vi "monitor.vi"() -> ()   [LabVIEW 2012]
uses:
  <vilib>/addons/database/Auxilliary.llb/DB Tools Cursor Type.ctl
  <vilib>/addons/database/Connection.llb/DB Tools Open Connec (Path).vi
  <vilib>/addons/database/Connection.llb/Conn Execute.vi
  <vilib>/addons/database/Recordset.llb/Rec Fetch Recordset Data (R).vi
  <vilib>/addons/database/Recordset.llb/Rec Destroy - Connection.vi
  <vilib>/addons/database/_DB Variant To Data/Database Variant To Data.xnode
  <vilib>/addons/database/NI_Database_API.lvlib
panel:
  in  "Table Control":string[][](table)
  out "error out 2":errorcluster
  in  "input cluster 2":T1
  in  "stop":bool
  in  "OK Button":bool
  in  "M100 Monitor Board":string[][](table)
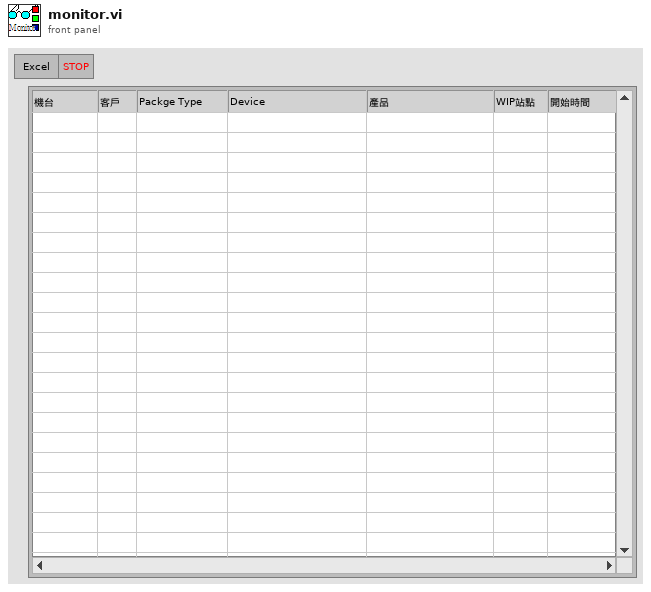
[diagram p1: front panel]
types:
  T1 = cluster{"Customer":string, "Package":string, "machine":string}
  T2 = typedef "NI_Database_API.lvlib/DB Tools Cursor Type.ctl" = enum16{"forward-only", "keyset", "dynamic", "static"}
  T3 = typedef "NI_Database_API.lvlib/Conn ObjectReference.ctl" = refnum<k1>
  T4 = typedef "LVDateTimeRec.ctl" = cluster{"fractional second":dbl, "second":i32, "minute":i32, "hour":i32, "day of month":i32, "month":i32, "year":i32, "day of week":i32, "day of year":i32, "DST":i32}
  T5 = typedef "LVRowAndColumnTypeDef.ctl" = cluster{"Row":i32, "Column":i32}
  T6 = typedef "NI_Database_API.lvlib/Rec ObjectReference.ctl" = refnum<k1>
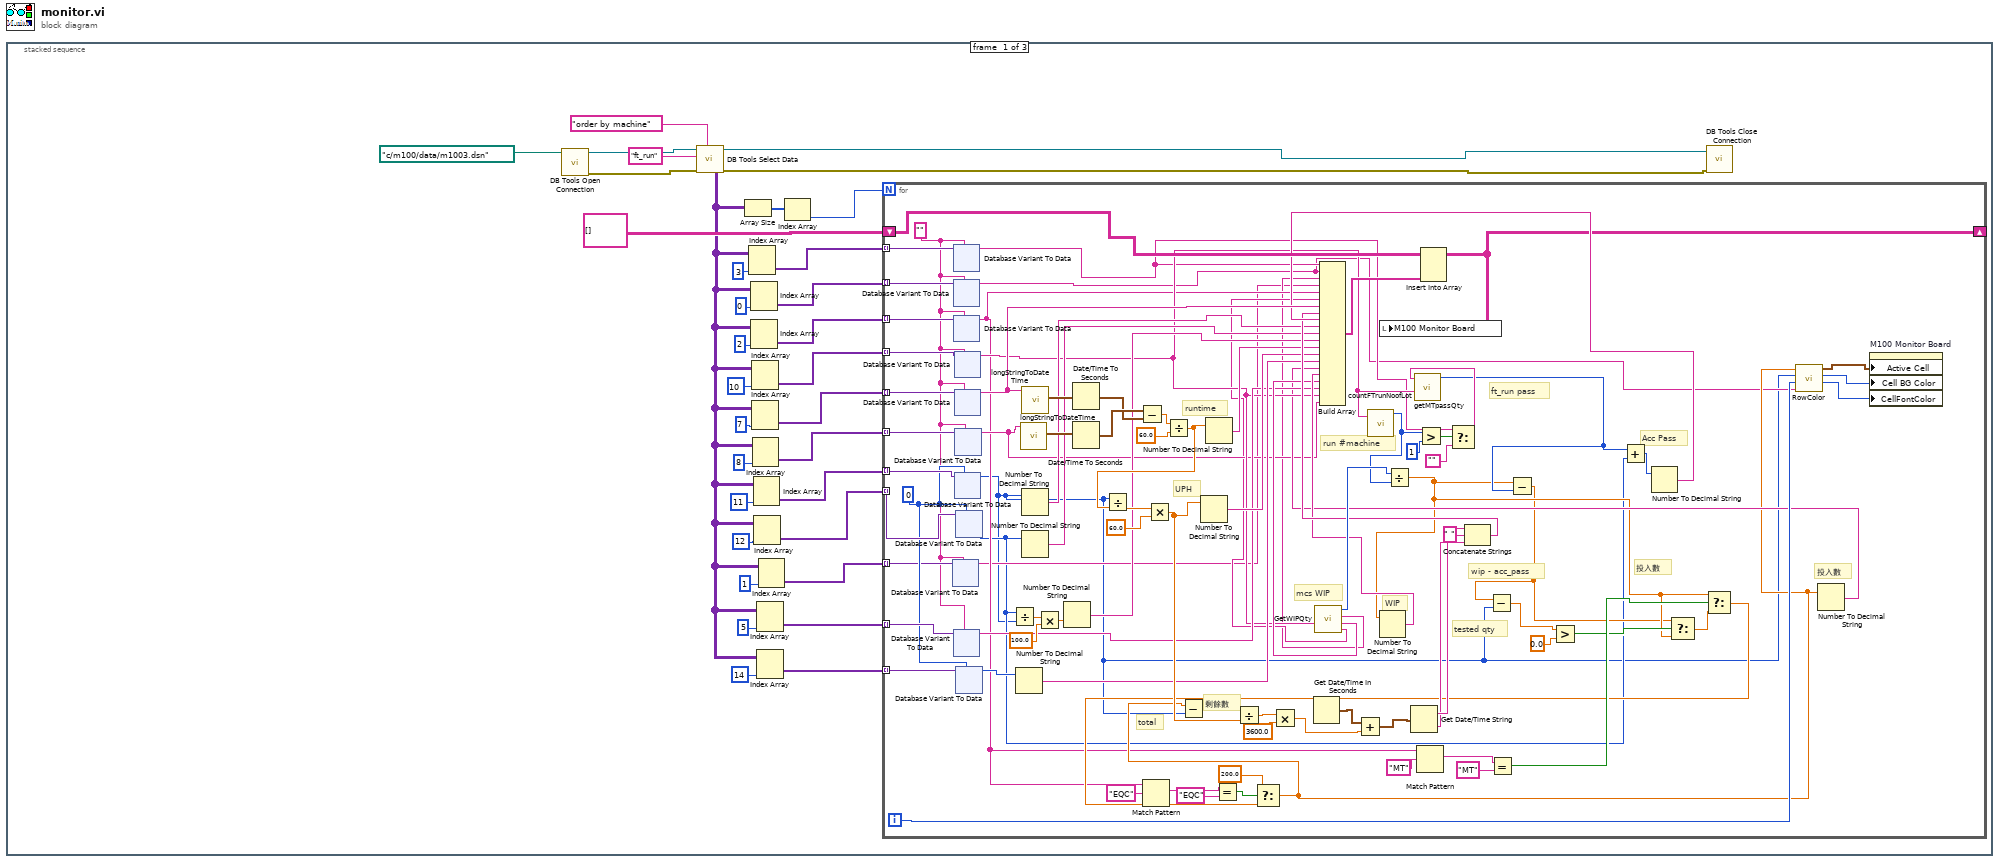
[diagram p0: block diagram]
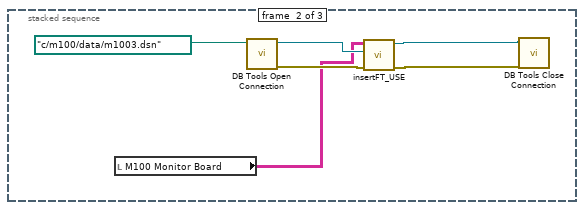
[diagram p2: hidden frame]
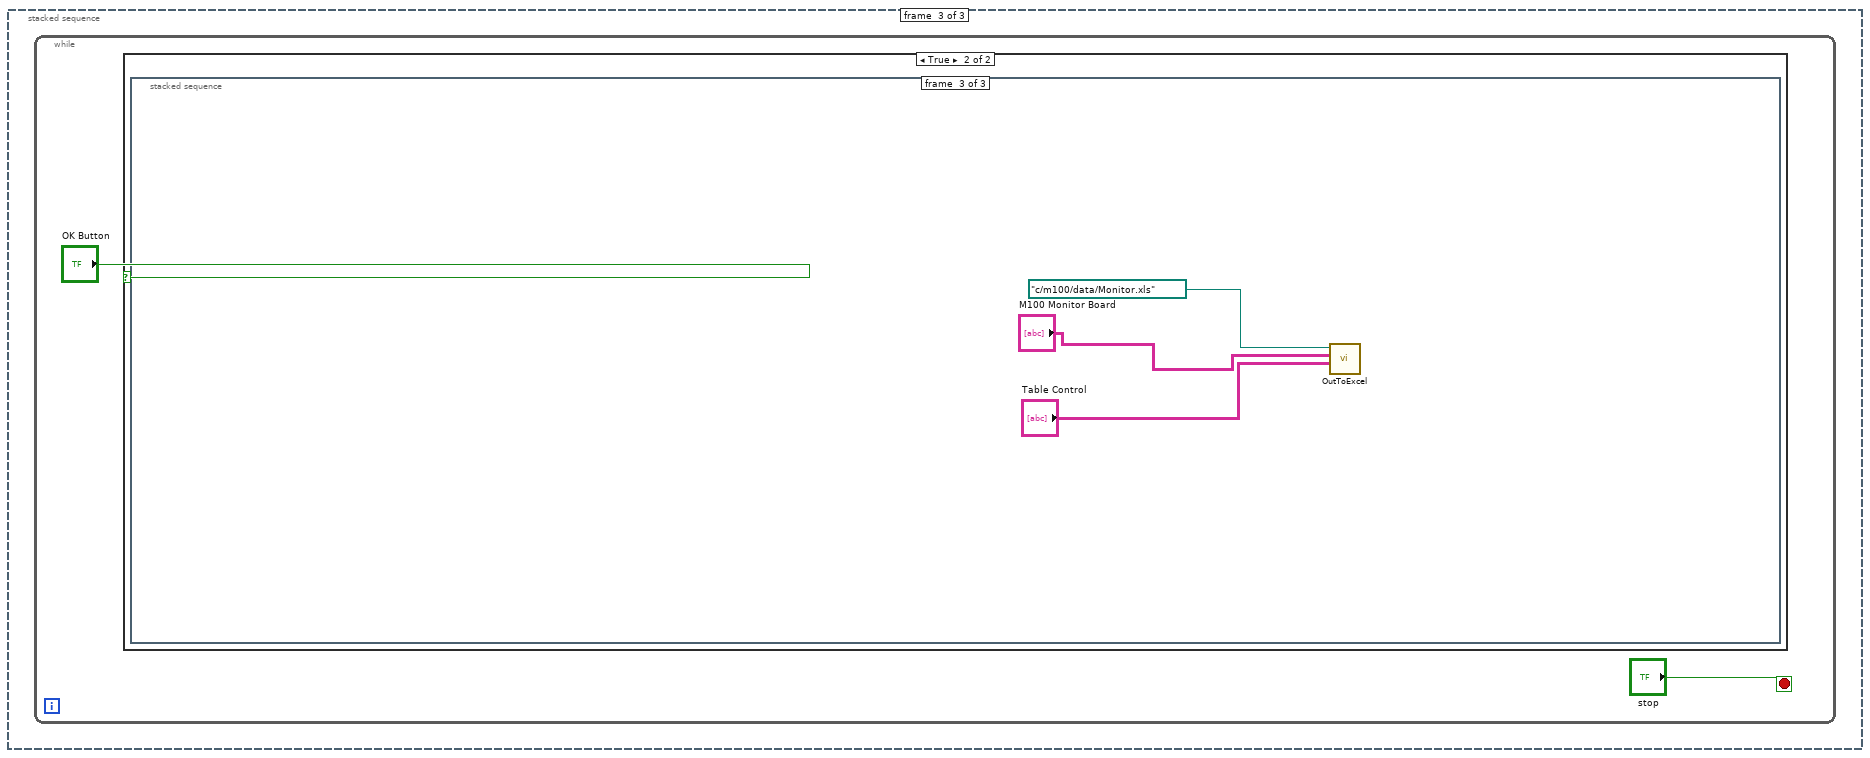
[diagram p3: hidden frame]
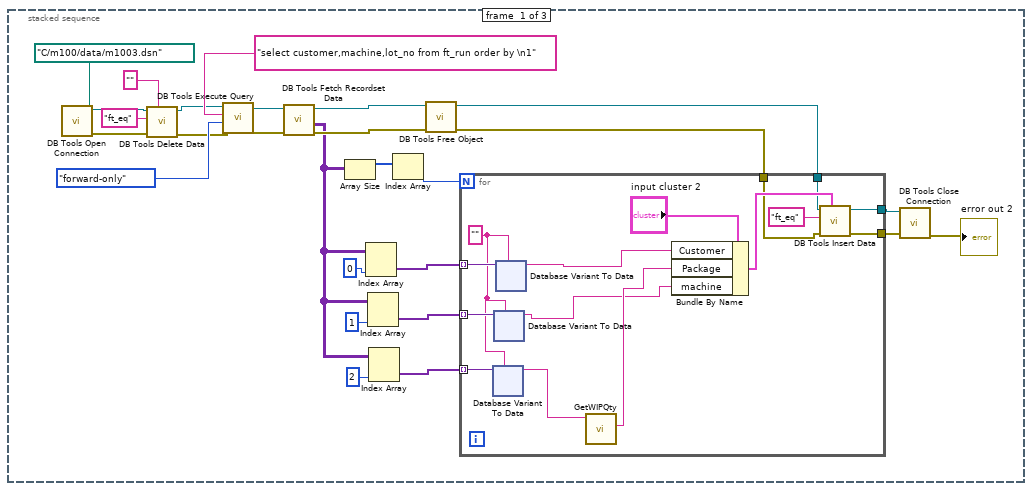
[diagram p5: hidden frame]
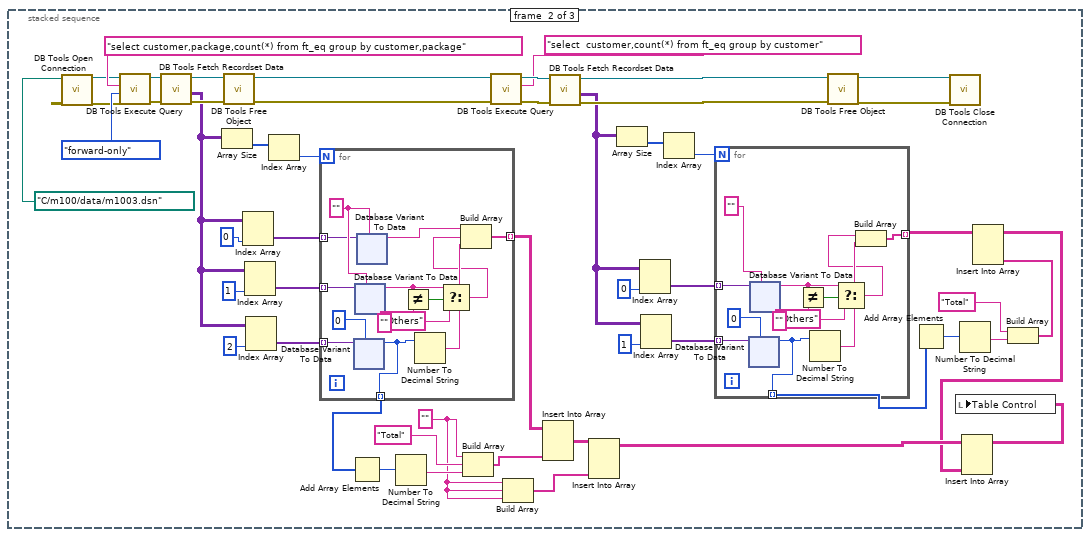
[diagram p6: hidden frame]
diagram:
  n1 = stacked-sequence {
    frame #0 {
      n2 = call-poly <vilib>:"DB Tools Open Connection.vi"("connection information"=path "c:/m100/data/m1003.dsn") -> ("error out"=w32:errorcluster, "connection reference"=w33:T3)  [unwired: 7 in]
      n3 = call <vilib>:"DB Tools Select Data.vi"("condition"="order by machine", "error in (no error)"=w32, "table"="ft_run", "connection reference"=w33) -> ("error out"=w1:errorcluster, "data"=w5:variant[][], "connection reference out"=w2:T3)  [unwired: 2 in]
      n4 = Array Size(array=w5) -> (size(s)=w29:i32[])
      n5 = Index Array(array=w5, index (col)=3) -> (element=w18:variant[])  [unwired: 1 in]
      n6 = Index Array(array=w5, index (col)=0) -> (element=w25:variant[])  [unwired: 1 in]
      n7 = Index Array(array=w5, index (col)=2) -> (element=w17:variant[])  [unwired: 1 in]
      n8 = Index Array(array=w5, index (col)=10) -> (element=w16:variant[])  [unwired: 1 in]
      n9 = Index Array(array=w5, index (col)=7) -> (element=w15:variant[])  [unwired: 1 in]
      n10 = Index Array(array=w5, index (col)=8) -> (element=w11:variant[])  [unwired: 1 in]
      n11 = Index Array(array=w5, index (col)=11) -> (element=w14:variant[])  [unwired: 1 in]
      n12 = Index Array(array=w5, index (col)=12) -> (element=w13:variant[])  [unwired: 1 in]
      n13 = Index Array(array=w5, index (col)=5) -> (element=w9:variant[])  [unwired: 1 in]
      n14 = Index Array(array=w5, index (col)=14 ("disabled index (col)")) -> (element=w7:variant[])  [unwired: 1 in]
      n15 = Index Array(array=w5, index (col)=1 ("disabled index (col)")) -> (element=w3:variant[])  [unwired: 1 in]
      n16 = Index Array(array=w29) -> (element=w28:i32)  [unwired: 1 in]
      n17 = for {
        N: w28 -> [_]
        tunnel: w25 -> [w120] mode=indexing
        tunnel: w13 -> [w124] mode=indexing
        shift-right: [w42] -> _
        shift-left: string[][] [] -> [w123]
        tunnel: w18 -> [w121] mode=indexing
        tunnel: w17 -> [w119] mode=indexing
        tunnel: w16 -> [w118] mode=indexing
        tunnel: w15 -> [w117] mode=indexing
        tunnel: w14 -> [w116] mode=indexing
        tunnel: w11 -> [w112] mode=indexing
        tunnel: w9 -> [w102] mode=indexing
        tunnel: w7 -> [w101] mode=indexing
        tunnel: w3 -> [w50] mode=indexing
        i -> [w86]
        w100 = 0
        w49 = ""
        # "tested qty"
        # "wip - acc_pass"
        # "投入數"
        # "剩餘數"
        # "ft_run pass"
        # "WIP"
        # "mcs WIP"
        # "run #machine"
        # "Acc Pass"
        # "total"
        # "UPH"
        # "runtime"
        # "投入數"
        n18 = xnode "Database Variant To Data"("database variant"=w50, "type"=w49) -> ("data"=w43:string)  [unwired: 1 in, 1 out]
        n19 = xnode "Database Variant To Data"("database variant"=w121, "type"=w49) -> ("data"=w46:string)  [unwired: 1 in, 1 out]
        n20 = xnode "Database Variant To Data"("database variant"=w120, "type"=w49) -> ("data"=w45:string)  [unwired: 1 in, 1 out]
        n21 = xnode "Database Variant To Data"("database variant"=w119, "type"=w49) -> ("data"=w48:string)  [unwired: 1 in, 1 out]
        n22 = xnode "Database Variant To Data"("database variant"=w102, "type"=w49) -> ("data"=w67:string)  [unwired: 1 in, 1 out]
        n23 = xnode "Database Variant To Data"("database variant"=w118, "type"=w49) -> ("data"=w66:string)  [unwired: 1 in, 1 out]
        n24 = xnode "Database Variant To Data"("database variant"=w117, "type"=w49) -> ("data"=w78:string)  [unwired: 1 in, 1 out]
        n25 = xnode "Database Variant To Data"("database variant"=w116, "type"=w100) -> ("data"=w34:i32)  [unwired: 1 in, 1 out]
        n26 = xnode "Database Variant To Data"("database variant"=w112, "type"=w49) -> ("data"=w63:string)  [unwired: 1 in, 1 out]
        n27 = xnode "Database Variant To Data"("database variant"=w124, "type"=w100) -> ("data"=w36:i32)  [unwired: 1 in, 1 out]
        n28 = xnode "Database Variant To Data"("database variant"=w101, "type"=w100) -> ("data"=w99:i32)  [unwired: 1 in, 1 out]
        n29 = Divide(x=w36, y=w34) -> (x/y=w113:dbl)
        n30 = Number To Decimal String(number=w99) -> (decimal integer string=w70:string)  [unwired: 1 in]
        n31 = call "longStringToDateTime.vi"("input string"=w63) -> ("output cluster"=w111:T4)  [unwired: 10 in]
        n32 = call "longStringToDateTime.vi"("input string"=w78) -> ("output cluster"=w110:T4)  [unwired: 10 in]
        n33 = Number To Decimal String(number=w34) -> (decimal integer string=w75:string)  [unwired: 1 in]
        n34 = Number To Decimal String(number=w36) -> (decimal integer string=w74:string)  [unwired: 1 in]
        n35 = Multiply(x=w113, y=100.0) -> (x*y=w114:dbl)
        n36 = Number To Decimal String(number=w114) -> (decimal integer string=w73:string)  [unwired: 1 in]
        n37 = Date/Time To Seconds(2:w110) -> (0:w108:timestamp)  [unwired: 1 in]
        n38 = Date/Time To Seconds(2:w111) -> (0:w109:timestamp)  [unwired: 1 in]
        n39 = Subtract(x=w109, y=w108) -> (x-y=w107:dbl)
        n40 = Match Pattern(string=w48, regular expression="EQC") -> (match substring=w61:string)  [unwired: 1 in, 3 out]
        n41 = Divide(x=w107, y=60.0) -> (x/y=w105:dbl)
        n42 = Divide(x=w34, y=w105) -> (x/y=w104:dbl)
        n43 = Multiply(x=w104, y=60.0) -> (x*y=w98:dbl)
        n44 = Number To Decimal String(number=w98) -> (decimal integer string=w71:string)  [unwired: 1 in]
        n45 = Number To Decimal String(number=w105) -> (decimal integer string=w72:string)  [unwired: 1 in]
        n46 = Equal?(x=w61, y="EQC") -> (x = y?=w59:bool)
        n47 = Get Date/Time In Seconds() -> (seconds since 1Jan1904=w95:timestamp)
        n48 = call "GetWIPQty.vi"("Lotno"=w66) -> ("step"=w47:string, "lotno"=w68:string, "Package"=w44:string, "data"=w85:i32)  [unwired: 7 in]
        n49 = call "countFTrunNoofLot.vi"("Lotno"=w66) -> ("data"=w83:i32)  [unwired: 10 in]
        n50 = Divide(x=w85, y=w83) -> (x/y=w39:dbl)
        n51 = Number To Decimal String(number=w39) -> (decimal integer string=w69:string)  [unwired: 1 in]
        n52 = Match Pattern(string=w48, regular expression="MT") -> (match substring=w56:string)  [unwired: 1 in, 3 out]
        n53 = Greater?(x=w83, y=1) -> (0:w81:bool)
        n54 = Select(t=w46, s=w81, f="") -> (s? t:f=w79:string)
        n55 = call "getMTpassQty.vi"("Lot"=w66, "machine"=w79) -> ("data"=w64:i32)  [unwired: 9 in]
        n56 = Equal?(x=w56, y="MT") -> (x = y?=w54:bool)
        n57 = Subtract(x=w39, y=w64) -> (x-y=w37:dbl)
        n58 = Subtract(x=w37, y=w34) -> (x-y=w35:dbl)
        n59 = Greater?(x=w35, y=0.0) -> (0:w40:bool)
        n60 = Add(x=w64, y=w36) -> (x+y=w84:i32)
        n61 = Number To Decimal String(number=w84) -> (decimal integer string=w77:string)  [unwired: 1 in]
        n62 = Select(t=w37, s=w40, f=w39) -> (s? t:f=w38:dbl)
        n63 = Select(t=w39, s=w54, f=w38) -> (s? t:f=w53:dbl)
        n64 = Select(t=200.0, s=w59, f=w53) -> (s? t:f=w51:dbl)
        n65 = Subtract(x=w51, y=w34) -> (x-y=w52:dbl)
        n66 = Divide(x=w52, y=w98) -> (x/y=w97:dbl)
        n67 = Multiply(x=w97, y=3600.0) -> (x*y=w94:dbl)
        n68 = Add(x=w95, y=w94) -> (x+y=w93:timestamp)
        n69 = Get Date/Time String(seconds (now)=w93) -> (date string=w92:string, time string=w91:string)  [unwired: 2 in]
        n70 = Concatenate Strings(w92, " " ("string"), w91) -> (w76:string)
        n71 = call "RowColor.vi"("Customer"=w45, "Row"=w86, "tested"=w34, "Input"=w51) -> ("FontColor"=w87:u32, "bgcolor"=w88:u32, "ActiveCell"=w89:T5)  [unwired: 5 in]
        n72 = Number To Decimal String(number=w51) -> (decimal integer string=w65:string)  [unwired: 1 in]
        n73 = Build Array(w46, w45, w44, w43, w48, w47, w78, w76, w77, w75, w74, w73, w72, w71, w70, w65, w69, w68, w67, w66, w63) -> (w122:string[])
        n74 = Insert Into Array(array=w123, new element=w122) -> (w42:string[][])  [unwired: 2 in]
        n75 = local write "M100 Monitor Board"(w42) -> ()
        n76 = property on="M100 Monitor Board" class="Tbl (strict)"("Active Cell"=w89, "Cell BG Color"=w88, "CellFontColor"=w87) -> ()  [unwired: 2 in, 2 out]
      }
      n77 = call <vilib>:"DB Tools Close Connection.vi"("error in (no error)"=w1, "connection reference"=w2) -> ()  [unwired: 5 in, 1 out]
    }
    frame #1 {
      n78 = local read "M100 Monitor Board"() -> (w477:string[][])
      n79 = call-poly <vilib>:"DB Tools Open Connection.vi"("connection information"=path "c:/m100/data/m1003.dsn") -> ("error out"=w480:errorcluster, "connection reference"=w481:T3)  [unwired: 7 in]
      n80 = call "insertFT_USE.vi"("M100 Monitor Board"=w477, "connection reference"=w481, "error in (no error)"=w480) -> ("connection reference out"=w479:T3, "error out"=w478:errorcluster)  [unwired: 6 in]
      n81 = call <vilib>:"DB Tools Close Connection.vi"("error in (no error)"=w478, "connection reference"=w479) -> ()  [unwired: 5 in, 1 out]
    }
    frame #2 {
      n82 = while {
        stop <- "stop" stop-if-true
        n83 = case shown="True" "OK Button" {
          frame False {
          }
          frame True {
            n84 = stacked-sequence {
              frame #0 {
                n85 = call-poly <vilib>:"DB Tools Open Connection.vi"("connection information"=path "C:/m100/data/m1003.dsn") -> ("error out"=w495:errorcluster, "connection reference"=w496:T3)  [unwired: 7 in]
                n86 = call <vilib>:"DB Tools Delete Data.vi"("condition"="", "error in (no error)"=w495, "table"="ft_eq", "connection reference"=w496) -> ("error out"=w493:errorcluster, "connection reference out"=w492:T3)  [unwired: 6 in]
                n87 = call-poly <vilib>:"DB Tools Execute Query.vi"("error in (no error)"=w493, "cursor type"=DB_Tools_Cursor_Type."forward-only", "SQL query"="select customer,machine,lot_no from ft_run order by \n1", "connection reference"=w492) -> ("error out"=w508:errorcluster, "recordset reference"=w510:T6)  [unwired: 4 in]
                n88 = call-poly <vilib>:"DB Tools Fetch Recordset Data.vi"("error in (no error)"=w508, "recordset reference"=w510) -> ("error out"=w507:errorcluster, "recordset data"=w502:variant[][], "recordset reference out"=w509:T6)  [unwired: 3 in]
                n89 = Array Size(array=w502) -> (size(s)=w501:i32[])
                n90 = Index Array(array=w502, index (col)=0 ("disabled index (col)")) -> (element=w499:variant[])  [unwired: 1 in]
                n91 = Index Array(array=w502, index (col)=1 ("disabled index (col)")) -> (element=w498:variant[])  [unwired: 1 in]
                n92 = Index Array(array=w502, index (col)=2) -> (element=w497:variant[])  [unwired: 1 in]
                n93 = Index Array(array=w501) -> (element=w500:i32)  [unwired: 1 in]
                n94 = call-poly <vilib>:"DB Tools Free Object.vi"("error in (no error)"=w507, "recordset reference"=w509) -> ("error out"=w488:errorcluster, "connection reference"=w489:T3)  [unwired: 8 in]
                n95 = for {
                  N: w500 -> [_]
                  tunnel: w499 -> [w526] mode=indexing
                  tunnel: w498 -> [w525] mode=indexing
                  tunnel: w497 -> [w524] mode=indexing
                  tunnel: w489 -> [w515]
                  tunnel: w488 -> [w514]
                  tunnel: [w513] -> w487
                  tunnel: [w512] -> w486
                  w523 = ""
                  n96 = xnode "Database Variant To Data"("database variant"=w524, "type"=w523) -> ("data"=w522:string)  [unwired: 1 in, 1 out]
                  n97 = xnode "Database Variant To Data"("database variant"=w525, "type"=w523) -> ("data"=w517:string)  [unwired: 1 in, 1 out]
                  n98 = xnode "Database Variant To Data"("database variant"=w526, "type"=w523) -> ("data"=w519:string)  [unwired: 1 in, 1 out]
                  n99 = call "GetWIPQty.vi"("Lotno"=w522) -> ("Package"=w518:string)  [unwired: 7 in, 3 out]
                  n100 = Bundle By Name(cluster="input cluster 2", "Customer"=w519, "Package"=w518, "machine"=w517) -> (w516:T1)
                  n101 = call <vilib>:"DB Tools Insert Data.vi"("data"=w516, "error in (no error)"=w514, "table"="ft_eq", "connection reference"=w515) -> ("error out"=w512:errorcluster, "connection reference out"=w513:T3)  [unwired: 6 in]
                }
                n102 = call <vilib>:"DB Tools Close Connection.vi"("error in (no error)"=w486, "connection reference"=w487) -> ("error out"=→"error out 2":errorcluster)  [unwired: 5 in]
              }
              frame #1 {
                w632 = "" ("element")
                n103 = call-poly <vilib>:"DB Tools Open Connection.vi"("connection information"=path "C:/m100/data/m1003.dsn") -> ("error out"=w661:errorcluster, "connection reference"=w662:T3)  [unwired: 7 in]
                n104 = call-poly <vilib>:"DB Tools Execute Query.vi"("error in (no error)"=w661, "cursor type"=DB_Tools_Cursor_Type."forward-only", "SQL query"="select customer,package,count(*) from ft_eq group by customer,package", "connection reference"=w662) -> ("error out"=w671:errorcluster, "recordset reference"=w673:T6)  [unwired: 4 in]
                n105 = call-poly <vilib>:"DB Tools Fetch Recordset Data.vi"("error in (no error)"=w671, "recordset reference"=w673) -> ("error out"=w670:errorcluster, "recordset data"=w665:variant[][], "recordset reference out"=w672:T6)  [unwired: 3 in]
                n106 = Array Size(array=w665) -> (size(s)=w664:i32[])
                n107 = call-poly <vilib>:"DB Tools Free Object.vi"("error in (no error)"=w670, "recordset reference"=w672) -> ("error out"=w629:errorcluster, "connection reference"=w630:T3)  [unwired: 8 in]
                n108 = Index Array(array=w665, index (col)=0 ("disabled index (col)")) -> (element=w659:variant[])  [unwired: 1 in]
                n109 = Index Array(array=w665, index (col)=1 ("disabled index (col)")) -> (element=w658:variant[])  [unwired: 1 in]
                n110 = Index Array(array=w665, index (col)=2) -> (element=w657:variant[])  [unwired: 1 in]
                n111 = Index Array(array=w664) -> (element=w660:i32)  [unwired: 1 in]
                n112 = for {
                  N: w660 -> [_]
                  tunnel: w659 -> [w763] mode=indexing
                  tunnel: w658 -> [w762] mode=indexing
                  tunnel: w657 -> [w761] mode=indexing
                  tunnel: [w757] -> w652 mode=indexing
                  tunnel: [w751] -> w655 mode=indexing
                  w764 = ""
                  n113 = xnode "Database Variant To Data"("database variant"=w761, "type"=0) -> ("data"=w751:i32)  [unwired: 1 in, 1 out]
                  n114 = xnode "Database Variant To Data"("database variant"=w762, "type"=w764) -> ("data"=w754:string)  [unwired: 1 in, 1 out]
                  n115 = xnode "Database Variant To Data"("database variant"=w763, "type"=w764) -> ("data"=w759:string)  [unwired: 1 in, 1 out]
                  n116 = Not Equal?(x=w754, y="") -> (x != y?=w755:bool)
                  n117 = Number To Decimal String(number=w751) -> (decimal integer string=w758:string)  [unwired: 1 in]
                  n118 = Select(t=w754, s=w755, f="Others") -> (s? t:f=w752:string)
                  n119 = Build Array(w759, w752, w758) -> (w757:string[])
                }
                n120 = Add Array Elements(numeric array=w655) -> (sum=w656:i32)
                n121 = Number To Decimal String(number=w656) -> (decimal integer string=w654:string)  [unwired: 1 in]
                n122 = Build Array(w632, "Total" ("element"), w654) -> (w651:string[])
                n123 = call-poly <vilib>:"DB Tools Execute Query.vi"("error in (no error)"=w629, "SQL query"="select  customer,count(*) from ft_eq group by customer", "connection reference"=w630) -> ("error out"=w648:errorcluster, "recordset reference"=w650:T6)  [unwired: 5 in]
                n124 = Build Array(w632, w632, w632) -> (w631:string[])
                n125 = Insert Into Array(array=w652, new element=w651) -> (w633:string[][])  [unwired: 2 in]
                n126 = call-poly <vilib>:"DB Tools Fetch Recordset Data.vi"("error in (no error)"=w648, "recordset reference"=w650) -> ("error out"=w647:errorcluster, "recordset data"=w644:variant[][], "recordset reference out"=w649:T6)  [unwired: 3 in]
                n127 = Insert Into Array(array=w633, new element=w631) -> (w625:string[][])  [unwired: 2 in]
                n128 = Array Size(array=w644) -> (size(s)=w643:i32[])
                n129 = Index Array(array=w644, index (col)=0 ("disabled index (col)")) -> (element=w641:variant[])  [unwired: 1 in]
                n130 = Index Array(array=w644, index (col)=1) -> (element=w640:variant[])  [unwired: 1 in]
                n131 = Index Array(array=w643) -> (element=w642:i32)  [unwired: 1 in]
                n132 = for {
                  N: w642 -> [_]
                  tunnel: w641 -> [w685] mode=indexing
                  tunnel: w640 -> [w684] mode=indexing
                  tunnel: [w681] -> w635 mode=indexing
                  tunnel: [w675] -> w638 mode=indexing
                  n133 = xnode "Database Variant To Data"("database variant"=w684, "type"=0) -> ("data"=w675:i32)  [unwired: 1 in, 1 out]
                  n134 = xnode "Database Variant To Data"("database variant"=w685, "type"="") -> ("data"=w678:string)  [unwired: 1 in, 1 out]
                  n135 = Not Equal?(x=w678, y="") -> (x != y?=w679:bool)
                  n136 = Number To Decimal String(number=w675) -> (decimal integer string=w682:string)  [unwired: 1 in]
                  n137 = Select(t=w678, s=w679, f="Others") -> (s? t:f=w676:string)
                  n138 = Build Array(w676, w682) -> (w681:string[])
                }
                n139 = call-poly <vilib>:"DB Tools Free Object.vi"("error in (no error)"=w647, "recordset reference"=w649) -> ("error out"=w627:errorcluster, "connection reference"=w628:T3)  [unwired: 8 in]
                n140 = Add Array Elements(numeric array=w638) -> (sum=w639:i32)
                n141 = call <vilib>:"DB Tools Close Connection.vi"("error in (no error)"=w627, "connection reference"=w628) -> ()  [unwired: 5 in, 1 out]
                n142 = Number To Decimal String(number=w639) -> (decimal integer string=w637:string)  [unwired: 1 in]
                n143 = Build Array("Total" ("element"), w637) -> (w634:string[])
                n144 = Insert Into Array(array=w635, new element=w634) -> (w624:string[][])  [unwired: 2 in]
                n145 = Insert Into Array(array=w625, new element=w624) -> (w623:string[][])  [unwired: 2 in]
                n146 = local write "Table Control"(w623) -> ()
              }
              frame #2 {
                n147 = call "OutToExcel.vi"("Table Control"="Table Control", "Running"="M100 Monitor Board", "Report Template"=path "c:/m100/data/Monitor.xls") -> ()  [unwired: 9 in]
              }
            }
          }
        }
      }
    }
  }
